vi "Get Readout Modes.vi"(8 "error in (no error)":errorcluster, 11 "Hamamatsu Camera in":refnum<class "Hamamatsu Camera.lvclass">) -> (0 "error out":errorcluster, 3 "Hamamatsu Camera out":refnum<class "Hamamatsu Camera.lvclass">)   [LabVIEW 2023, in "Hamamatsu Camera.lvlib" / "Hamamatsu Camera.lvclass"]
uses:
  Hamamatsu Camera.lvclass
  C:/Program Files/National Instruments/LabVIEW 2023/vi.lib/ActorFramework/Actor/Actor.lvclass
  <vilib>/ActorFramework/Actor/Actor.lvclass/Actor.ctl
  Application Messages/Update Camera Modes Msg/Update Camera Modes Msg.lvclass/Update Camera Modes Msg.ctl
  <vilib>/ActorFramework/Message Enqueuer/Message Enqueuer.lvclass/Message Enqueuer.ctl
  <vilib>/ActorFramework/Message Enqueuer/Enqueue.vi
  Application Messages/Update Camera Modes Msg/Update Camera Modes Msg.lvclass
  C:/Program Files/National Instruments/LabVIEW 2023/vi.lib/ActorFramework/Message/Message.lvclass
  <vilib>/ActorFramework/Message Priority Queue/Priority Enqueue.vi
  <vilib>/ActorFramework/Actor/Actor.lvclass
  Hamamatsu Camera.lvlib
panel:
  out "Allowed scan modes":cluster{"String":string, "Number":i32}[](array[cluster])
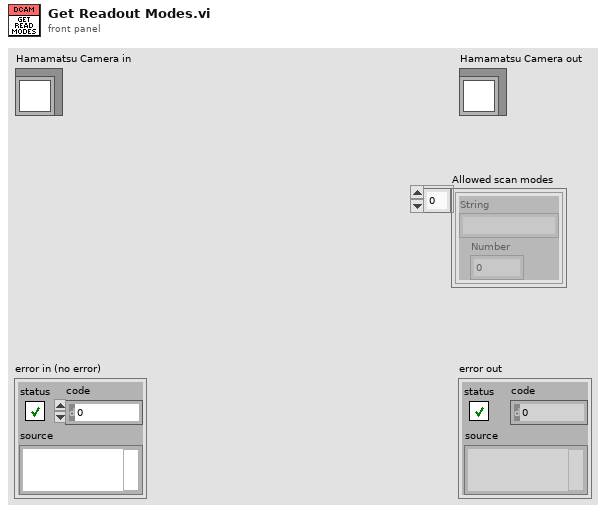
[diagram p1: front panel]
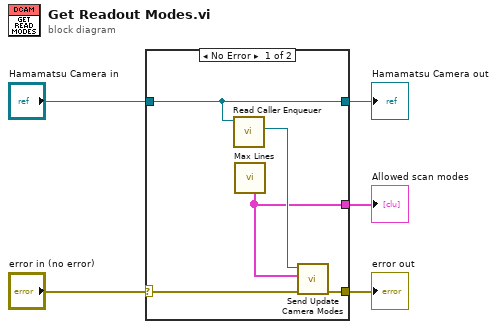
[diagram p0: block diagram]
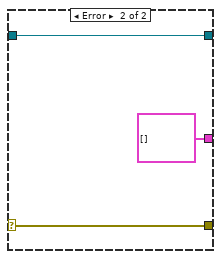
[diagram p2: hidden frame]
diagram:
  n1 = case shown="No Error" "error in (no error)" {
    selector: "error in (no error)" -> [w7 w13]
    tunnel: [w9 w13] -> w1
    tunnel: "Hamamatsu Camera in" -> [w8 w12]
    tunnel: [w8 w12] -> w2
    tunnel: [w6 cluster{"String":string, "Number":i32}[] [] ("Allowed scan modes")] -> w3
    frame No Error {
      n2 = call <vilib>:"Read Caller Enqueuer.vi"("Actor"=w8) -> ("Caller Enqueuer"=w10:refnum<class "Message Enqueuer.lvclass">)  [unwired: 10 in]
      n3 = call "Max Lines.vi"() -> ("Allowed scan modes"=w6:cluster{"String":string, "Value":i32}[])  [unwired: 6 in, 5 out]
      n4 = call "Send Update Camera Modes.vi"("error in (no error)"=w7, "StringsAndValues"=w6, "Message Enqueuer"=w10) -> ("error out"=w9:errorcluster)  [unwired: 7 in, 1 out]
    }
    frame Error {
    }
  }
  "error out" <- w1
  "Hamamatsu Camera out" <- w2
  "Allowed scan modes" <- w3
